vi "2015 Filepath Network Variable.vi"(5 "Network Var Set":u8, 7 "Washer In":T3={"Appliance Details"={"FileVersionInfo"={"FileVersion"="", "ProductName"="", "InternalName"="", "CompanyName"="", "LegalCopyright"="", "FileDescription"=""}, "Dishwasher Info"={"Open Cup Weight (gm):"=0.0, "Auto Cup Weight (gm):"=0.0, "Detergent-Dish:"="", "Inlet Temperature-Dish:"="", "Cycle Mode-Dish:"="", "Unit Control-Dish:"="", "Manufacturer-Dish:"=""}, "Washer Info"={"Hot Water Temperature (Fahrenheit):"="", "Cold Water Temperature (Fahrenheit):"="", "Capacity (cu.ft):"=0.0, "Initial Cloth Weight:"=0.0, "Cloth Lot:"=0, "Model Family:"="", "Program Name:"="", "Cycle Selection:"="", "Wash Temperature:"="", "Rinse Temperature:"="", "Load Size:"=""}, "File Name Output Array"=[], "Calibration Output Array"=[], "Appliance Common"={"Engineer:"="", "Model Number:"="", "Serial Number:"="", "Comments:"="", "Station ID:"="", "Technician:"="", "TR Number:"="", "Lab ID:"="", "Voltage:"="", "Water Pressure (PSI):"="", "Test Date:"="", "Computer Name:"="", "IP Address:"="", "Ambient RH:"="", "Frequency:"="", "Build:"="", "Filename:"="", "Test Type:"="", "Load Run #:"=0, "Ambient Temperature (F):"="", "File Path:"=path "", "Cycles Per Year"=60}, "Water Heater"={"Heating Mode:"=""}, "Dryer"={"Heat Setting:"="", "Washer Water Temperature (60 ± 5°F):"=60, "Water Hardness (PPM):"=17, "Dryness Setting:"="", "Dryer Type:"="", "Exhaust:"="", "Drying Cycle:"="", "Load Type:"="", "Nominal Load Weight"="", "Dryer Initial IMC Data"={"Measured IMC (lbs)"=7.0, "Actual Initial RMC (%)"=7.0, "RMC (Desired %)"=100.0, "Bone Dry Wt(lbs)"=7.0, "Tolerance(%)"=5.0, "Actual Final RMC (%)"=7.0, "CEF (lbf/kWh)"=0.0, "Minimum Weight (lbf)"=0.0, "Average Weight (lbf)"=0.0, "Maximum Weight (lbf)"=0.0, "Measured IMC In Range?"=FALSE, "Moisture Reduction Factor"=55.5, "Field Use Factor"=1.04, "Empty Dryer Cold Weigth"=0.0, "Energy Standard"=enum."D2-Automatic Dryer", "Weight Cloth (lbs)"=0.0, "Relative Moisture Content (%)"=0.0, "Relative Moisture Content - Avg (%)"=0.0}}}, "Display Data (RLT)"={"Status Color"=0, "Serial Number Display"="", "Cycle Count Display"=0, "Station Label Display"="", "Current Run Start Time Display"=0.0, "Board ID Display"="", "RPM Display"=0, "Current Display"=0.0, "Current Path Display"=path "", "Saving Display"=FALSE, "Unit Type Display"=enum."", "Total Time On Display"=0.0, "UI Button"=FALSE}} {"Display Data (RLT)"."Current Display" format="%.2f"; "Display Data (RLT)"."Cycle Count Display" format="%04d"; "Appliance Details"."Dryer"."Dryer Initial IMC Data"."Maximum Weight (lbf)" format="%03_6g"; "Appliance Details"."Dryer"."Dryer Initial IMC Data"."Average Weight (lbf)" format="%03_6g"; "Appliance Details"."Dryer"."Dryer Initial IMC Data"."Minimum Weight (lbf)" format="%03_6g"; "Appliance Details"."Dryer"."Dryer Initial IMC Data"."CEF (lbf/kWh)" format="%03_6g"; "Appliance Details"."Dryer"."Dryer Initial IMC Data"."Actual Final RMC (%)" format="%03_6g"; "Appliance Details"."Dryer"."Dryer Initial IMC Data"."Tolerance(%)" format="%0#_6g"; "Appliance Details"."Dryer"."Dryer Initial IMC Data"."Bone Dry Wt(lbs)" format="%03_6g"; "Appliance Details"."Dryer"."Dryer Initial IMC Data"."RMC (Desired %)" format="%0#_6g"; "Appliance Details"."Dryer"."Dryer Initial IMC Data"."Actual Initial RMC (%)" format="%03_6g"; "Appliance Details"."Dryer"."Dryer Initial IMC Data"."Measured IMC (lbs)" format="%0#_6g"}, 8 "error in (no error)":errorcluster, 10 "Network Variable Location":i32, 11 "File Locations In":T1={"General Setup Paths"={"Calibration File Path"=path "", "DOE Capacity Path"=path "", "Data Folder Path"=path "", "RLT Backup Data Path"=path "", "Tool Base Path"=path "", "General Startup Config Path"=path "", "File Save Previous Run Path"=path "", "File Save Configuration Data Path"=path "C:/Newfi Exe/Newfi Exe Locations.ini"}, "Data File Paths"={"Data File Path"=path "", "Debug File Path"=path "", "Bus Log Path"=path "", "Current"=path "", "Summary"=path ""}, "New Summary Created"=FALSE, "Check Location Interval (Second)"=2}) -> (0 "error out":errorcluster, 3 "File Locations Out":T1={"General Setup Paths"={"Calibration File Path"=path "", "DOE Capacity Path"=path "", "Data Folder Path"=path "", "RLT Backup Data Path"=path "", "Tool Base Path"=path "", "General Startup Config Path"=path "", "File Save Previous Run Path"=path "", "File Save Configuration Data Path"=path "C:/Newfi Exe/Newfi Exe Locations.ini"}, "Data File Paths"={"Data File Path"=path "", "Debug File Path"=path "", "Bus Log Path"=path "", "Current"=path "", "Summary"=path ""}, "New Summary Created"=FALSE, "Check Location Interval (Second)"=2})   [LabVIEW 2016]
uses:
  Utility/Save File/Public/Type Definitions/Save File Washer.ctl
  Utility/Save File/File Setup (Public)/Type Definition/Save File DISH Dishwasher Details.ctl
  <vilib>/Platform/fileVersionInfo.llb/FileVersionInformation.ctl
  Washer DOE/Type Definitions/DOE Appliance Common.ctl
  Utility/Custom Pallet Controls/Custom Pallet String.ctl
  Utility/Save File/File Setup (Public)/Type Definition/DPT IMC Data.ctl
  Washer DOE/Type Definitions/DOE Dryer Standard.ctl
  Utility/Save File/Public/Type Definitions/Save File Appliance Display.ctl
  Utility/Save File/Public/Type Definitions/Save File Unit Type.ctl
  Utility/Save File/File Setup (Public)/Type Definition/Save File DOE File Path Control.ctl
  Utility/Save File/File Setup (Public)/Type Definition/Save File DOE Data Save Filepaths.ctl
  Utility/Save File/Save File.lvlib
  Utility/Save File/File Setup.lvlib
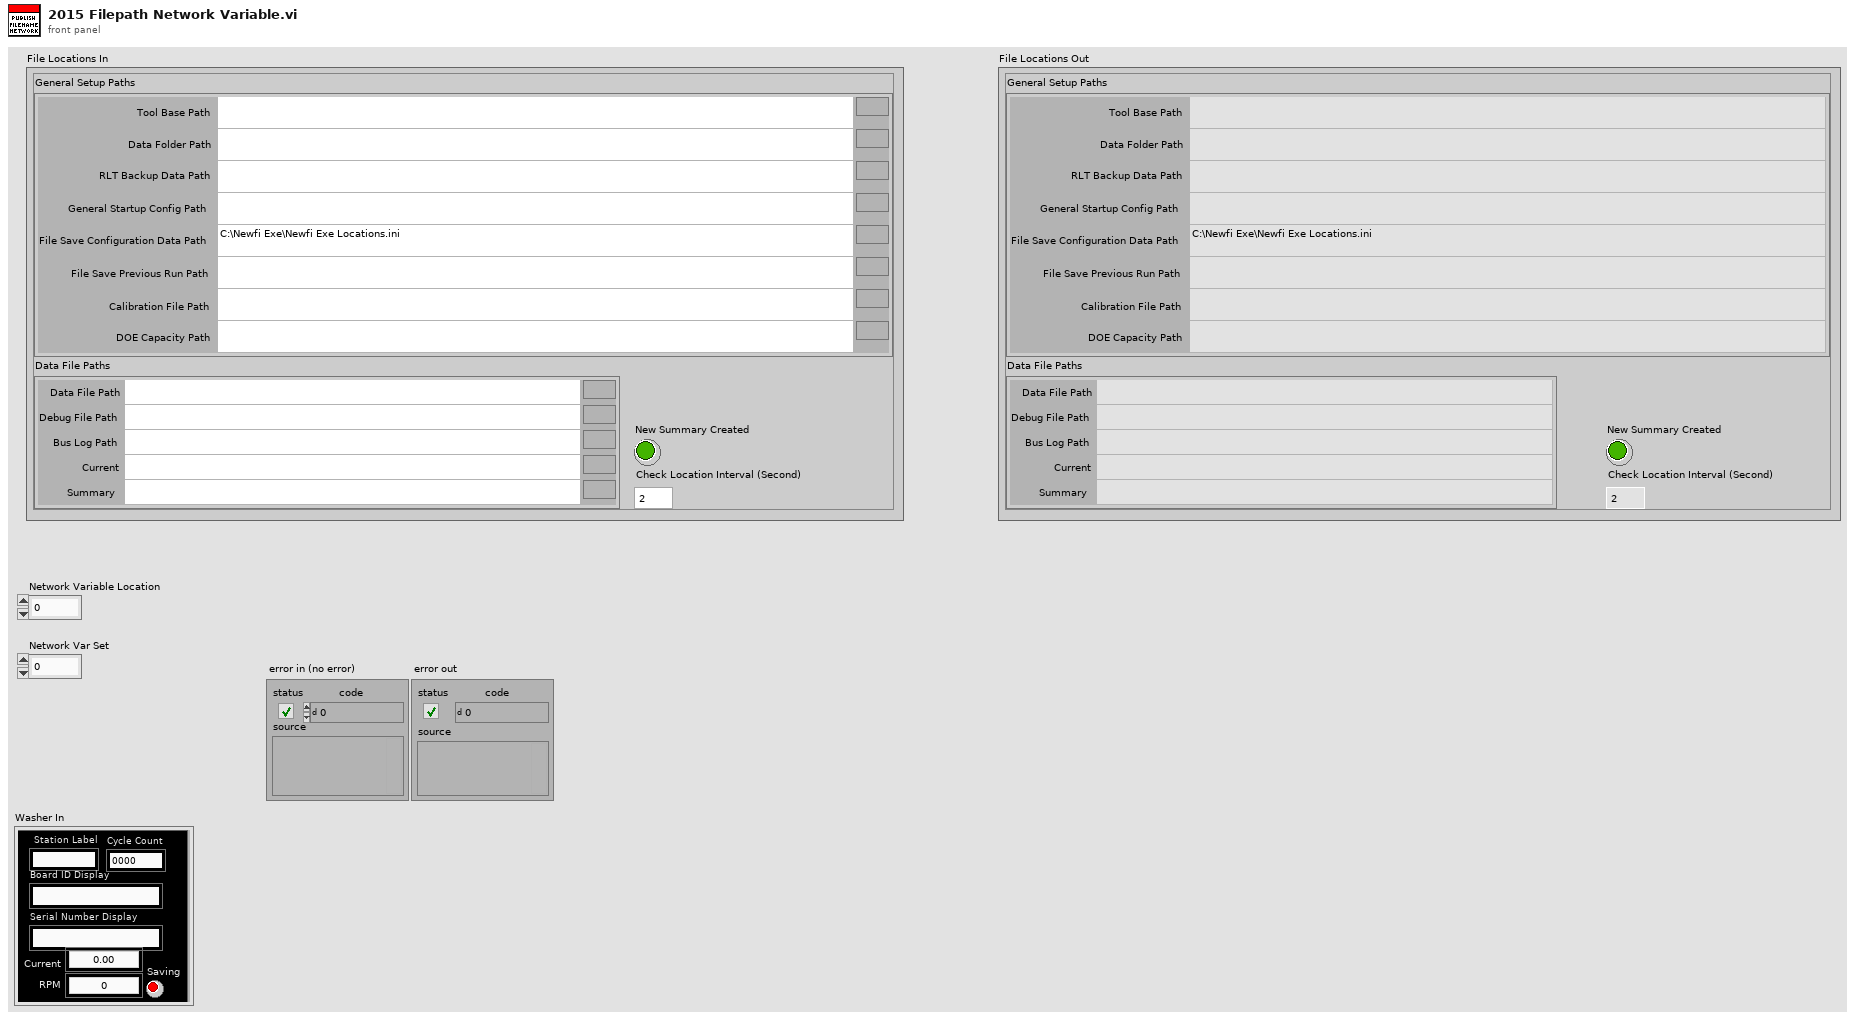
[diagram p1: front panel]
types:
  T1 = typedef "File Setup.lvlib/Save File DOE File Path Control.ctl" = cluster{"General Setup Paths":cluster{"Calibration File Path":path, "DOE Capacity Path":path, "Data Folder Path":path, "RLT Backup Data Path":path, "Tool Base Path":path, "General Startup Config Path":path, "File Save Previous Run Path":path, "File Save Configuration Data Path":path}, "Data File Paths":T2, "New Summary Created":bool, "Check Location Interval (Second)":i32}
  T2 = typedef "File Setup.lvlib/Save File DOE Data Save Filepaths.ctl" = cluster{"Data File Path":path, "Debug File Path":path, "Bus Log Path":path, "Current":path, "Summary":path}
  T3 = typedef "Save File.lvlib/Save File Washer.ctl" = cluster{"Appliance Details":T4, "Display Data (RLT)":T10}
  T4 = typedef "File Setup.lvlib/Save File DISH Dishwasher Details.ctl" = cluster{"FileVersionInfo":T5, "Dishwasher Info":cluster{"Open Cup Weight (gm):":dbl, "Auto Cup Weight (gm):":dbl, "Detergent-Dish:":string, "Inlet Temperature-Dish:":string, "Cycle Mode-Dish:":string, "Unit Control-Dish:":string, "Manufacturer-Dish:":string}, "Washer Info":cluster{"Hot Water Temperature (Fahrenheit):":string, "Cold Water Temperature (Fahrenheit):":string, "Capacity (cu.ft):":dbl, "Initial Cloth Weight:":dbl, "Cloth Lot:":i32, "Model Family:":string, "Program Name:":string, "Cycle Selection:":string, "Wash Temperature:":string, "Rinse Temperature:":string, "Load Size:":string}, "File Name Output Array":string[][], "Calibration Output Array":string[][], "Appliance Common":T6, "Water Heater":cluster{"Heating Mode:":string}, "Dryer":cluster{"Heat Setting:":T7, "Washer Water Temperature (60 ± 5°F):":u16, "Water Hardness (PPM):":u16, "Dryness Setting:":T7, "Dryer Type:":string, "Exhaust:":string, "Drying Cycle:":string, "Load Type:":string, "Nominal Load Weight":string, "Dryer Initial IMC Data":T8}}
  T5 = typedef "FileVersionInformation.ctl" = cluster{"FileVersion":string, "ProductName":string, "InternalName":string, "CompanyName":string, "LegalCopyright":string, "FileDescription":string}
  T6 = typedef "DOE Appliance Common.ctl" = cluster{"Engineer:":string, "Model Number:":string, "Serial Number:":string, "Comments:":string, "Station ID:":string, "Technician:":string, "TR Number:":string, "Lab ID:":string, "Voltage:":string, "Water Pressure (PSI):":string, "Test Date:":string, "Computer Name:":string, "IP Address:":string, "Ambient RH:":string, "Frequency:":string, "Build:":string, "Filename:":string, "Test Type:":string, "Load Run #:":i32, "Ambient Temperature (F):":string, "File Path:":path, "Cycles Per Year":u32}
  T7 = typedef "Custom Pallet String.ctl" = string
  T8 = typedef "DPT IMC Data.ctl" = cluster{"Measured IMC (lbs)":dbl, "Actual Initial RMC (%)":dbl, "RMC (Desired %)":dbl, "Bone Dry Wt(lbs)":dbl, "Tolerance(%)":dbl, "Actual Final RMC (%)":dbl, "CEF (lbf/kWh)":dbl, "Minimum Weight (lbf)":dbl, "Average Weight (lbf)":dbl, "Maximum Weight (lbf)":dbl, "Measured IMC In Range?":bool, "Moisture Reduction Factor":dbl, "Field Use Factor":dbl, "Empty Dryer Cold Weigth":dbl, "Energy Standard":T9, "Weight Cloth (lbs)":dbl, "Relative Moisture Content (%)":dbl, "Relative Moisture Content - Avg (%)":dbl}
  T9 = typedef "DOE Dryer Standard.ctl" = enum16{"D2-Automatic Dryer", "D2-Timer Dryer", "D1-Automatic Dryer", "D1-Timer Dryer", "Other"}
  T10 = typedef "Save File Appliance Display.ctl" = cluster{"Status Color":u32, "Serial Number Display":string, "Cycle Count Display":i32, "Station Label Display":string, "Current Run Start Time Display":dbl, "Board ID Display":string, "RPM Display":u32, "Current Display":dbl, "Current Path Display":path, "Saving Display":bool, "Unit Type Display":T11, "Total Time On Display":dbl, "UI Button":bool}
  T11 = typedef "Save File.lvlib/Save File Unit Type.ctl" = enum32{"", "Viper", "Hawk", "2015"}
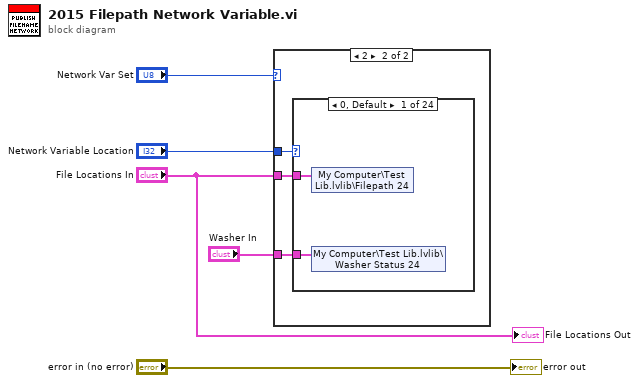
[diagram p0: block diagram]
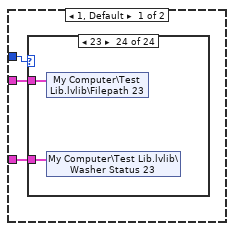
[diagram p2: hidden frame]
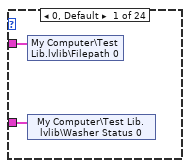
[diagram p3: hidden frame]
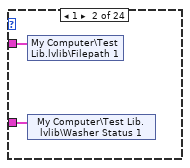
[diagram p4: hidden frame]
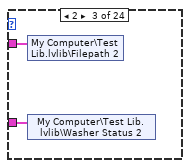
[diagram p5: hidden frame]
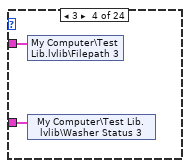
[diagram p6: hidden frame]
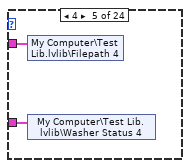
[diagram p7: hidden frame]
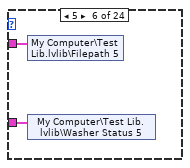
[diagram p8: hidden frame]
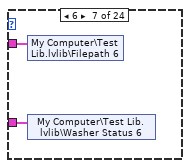
[diagram p9: hidden frame]
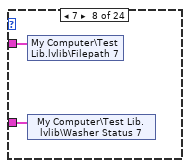
[diagram p10: hidden frame]
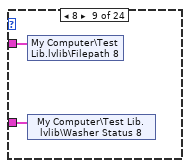
[diagram p11: hidden frame]
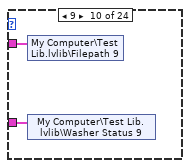
[diagram p12: hidden frame]
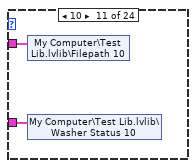
[diagram p13: hidden frame]
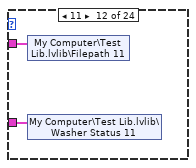
[diagram p14: hidden frame]
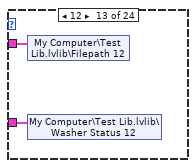
[diagram p15: hidden frame]
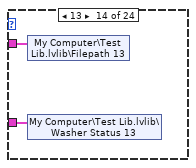
[diagram p16: hidden frame]
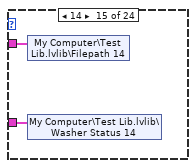
[diagram p17: hidden frame]
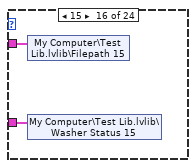
[diagram p18: hidden frame]
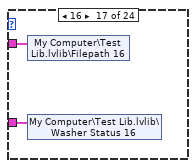
[diagram p19: hidden frame]
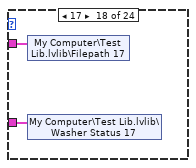
[diagram p20: hidden frame]
diagram:
  n1 = case shown="2" "Network Var Set" {
    tunnel: "File Locations In" -> [w8 w58]
    tunnel: "Network Variable Location" -> [w7 w57]
    tunnel: "Washer In" -> [w6 w59]
    frame 1, Default {
      n2 = case shown="23" w7 {
        tunnel: w8 -> [w10 w12 w14 w16 w18 w20 w22 w24 w26 w28 w30 w32 w34 w36 w38 w40 w42 w44 w46 w48 w50 w52 w54 w56]
        tunnel: w6 -> [w9 w11 w13 w15 w17 w19 w21 w23 w25 w27 w29 w31 w33 w35 w37 w39 w41 w43 w45 w47 w49 w51 w53 w55]
        frame 0, Default {
          n3 = shared-variable "My Computer\\Test Lib.lvlib\\Filepath 0"(w10) -> ()  [unwired: 1 in, 1 out]
          n4 = shared-variable "My Computer\\Test Lib.lvlib\\Washer Status 0"(w9) -> ()  [unwired: 1 in, 1 out]
        }
        frame 1 {
          n5 = shared-variable "My Computer\\Test Lib.lvlib\\Filepath 1"(w12) -> ()  [unwired: 1 in, 1 out]
          n6 = shared-variable "My Computer\\Test Lib.lvlib\\Washer Status 1"(w11) -> ()  [unwired: 1 in, 1 out]
        }
        frame 2 {
          n7 = shared-variable "My Computer\\Test Lib.lvlib\\Filepath 2"(w14) -> ()  [unwired: 1 in, 1 out]
          n8 = shared-variable "My Computer\\Test Lib.lvlib\\Washer Status 2"(w13) -> ()  [unwired: 1 in, 1 out]
        }
        frame 3 {
          n9 = shared-variable "My Computer\\Test Lib.lvlib\\Filepath 3"(w16) -> ()  [unwired: 1 in, 1 out]
          n10 = shared-variable "My Computer\\Test Lib.lvlib\\Washer Status 3"(w15) -> ()  [unwired: 1 in, 1 out]
        }
        frame 4 {
          n11 = shared-variable "My Computer\\Test Lib.lvlib\\Filepath 4"(w18) -> ()  [unwired: 1 in, 1 out]
          n12 = shared-variable "My Computer\\Test Lib.lvlib\\Washer Status 4"(w17) -> ()  [unwired: 1 in, 1 out]
        }
        frame 5 {
          n13 = shared-variable "My Computer\\Test Lib.lvlib\\Filepath 5"(w20) -> ()  [unwired: 1 in, 1 out]
          n14 = shared-variable "My Computer\\Test Lib.lvlib\\Washer Status 5"(w19) -> ()  [unwired: 1 in, 1 out]
        }
        frame 6 {
          n15 = shared-variable "My Computer\\Test Lib.lvlib\\Filepath 6"(w22) -> ()  [unwired: 1 in, 1 out]
          n16 = shared-variable "My Computer\\Test Lib.lvlib\\Washer Status 6"(w21) -> ()  [unwired: 1 in, 1 out]
        }
        frame 7 {
          n17 = shared-variable "My Computer\\Test Lib.lvlib\\Filepath 7"(w24) -> ()  [unwired: 1 in, 1 out]
          n18 = shared-variable "My Computer\\Test Lib.lvlib\\Washer Status 7"(w23) -> ()  [unwired: 1 in, 1 out]
        }
        frame 8 {
          n19 = shared-variable "My Computer\\Test Lib.lvlib\\Filepath 8"(w26) -> ()  [unwired: 1 in, 1 out]
          n20 = shared-variable "My Computer\\Test Lib.lvlib\\Washer Status 8"(w25) -> ()  [unwired: 1 in, 1 out]
        }
        frame 9 {
          n21 = shared-variable "My Computer\\Test Lib.lvlib\\Filepath 9"(w28) -> ()  [unwired: 1 in, 1 out]
          n22 = shared-variable "My Computer\\Test Lib.lvlib\\Washer Status 9"(w27) -> ()  [unwired: 1 in, 1 out]
        }
        frame 10 {
          n23 = shared-variable "My Computer\\Test Lib.lvlib\\Filepath 10"(w30) -> ()  [unwired: 1 in, 1 out]
          n24 = shared-variable "My Computer\\Test Lib.lvlib\\Washer Status 10"(w29) -> ()  [unwired: 1 in, 1 out]
        }
        frame 11 {
          n25 = shared-variable "My Computer\\Test Lib.lvlib\\Filepath 11"(w32) -> ()  [unwired: 1 in, 1 out]
          n26 = shared-variable "My Computer\\Test Lib.lvlib\\Washer Status 11"(w31) -> ()  [unwired: 1 in, 1 out]
        }
        frame 12 {
          n27 = shared-variable "My Computer\\Test Lib.lvlib\\Filepath 12"(w34) -> ()  [unwired: 1 in, 1 out]
          n28 = shared-variable "My Computer\\Test Lib.lvlib\\Washer Status 12"(w33) -> ()  [unwired: 1 in, 1 out]
        }
        frame 13 {
          n29 = shared-variable "My Computer\\Test Lib.lvlib\\Filepath 13"(w36) -> ()  [unwired: 1 in, 1 out]
          n30 = shared-variable "My Computer\\Test Lib.lvlib\\Washer Status 13"(w35) -> ()  [unwired: 1 in, 1 out]
        }
        frame 14 {
          n31 = shared-variable "My Computer\\Test Lib.lvlib\\Filepath 14"(w38) -> ()  [unwired: 1 in, 1 out]
          n32 = shared-variable "My Computer\\Test Lib.lvlib\\Washer Status 14"(w37) -> ()  [unwired: 1 in, 1 out]
        }
        frame 15 {
          n33 = shared-variable "My Computer\\Test Lib.lvlib\\Filepath 15"(w40) -> ()  [unwired: 1 in, 1 out]
          n34 = shared-variable "My Computer\\Test Lib.lvlib\\Washer Status 15"(w39) -> ()  [unwired: 1 in, 1 out]
        }
        frame 16 {
          n35 = shared-variable "My Computer\\Test Lib.lvlib\\Filepath 16"(w42) -> ()  [unwired: 1 in, 1 out]
          n36 = shared-variable "My Computer\\Test Lib.lvlib\\Washer Status 16"(w41) -> ()  [unwired: 1 in, 1 out]
        }
        frame 17 {
          n37 = shared-variable "My Computer\\Test Lib.lvlib\\Filepath 17"(w44) -> ()  [unwired: 1 in, 1 out]
          n38 = shared-variable "My Computer\\Test Lib.lvlib\\Washer Status 17"(w43) -> ()  [unwired: 1 in, 1 out]
        }
        frame 18 {
          n39 = shared-variable "My Computer\\Test Lib.lvlib\\Filepath 18"(w46) -> ()  [unwired: 1 in, 1 out]
          n40 = shared-variable "My Computer\\Test Lib.lvlib\\Washer Status 18"(w45) -> ()  [unwired: 1 in, 1 out]
        }
        frame 19 {
          n41 = shared-variable "My Computer\\Test Lib.lvlib\\Filepath 19"(w48) -> ()  [unwired: 1 in, 1 out]
          n42 = shared-variable "My Computer\\Test Lib.lvlib\\Washer Status 19"(w47) -> ()  [unwired: 1 in, 1 out]
        }
        frame 20 {
          n43 = shared-variable "My Computer\\Test Lib.lvlib\\Filepath 20"(w50) -> ()  [unwired: 1 in, 1 out]
          n44 = shared-variable "My Computer\\Test Lib.lvlib\\Washer Status 20"(w49) -> ()  [unwired: 1 in, 1 out]
        }
        frame 21 {
          n45 = shared-variable "My Computer\\Test Lib.lvlib\\Filepath 21"(w52) -> ()  [unwired: 1 in, 1 out]
          n46 = shared-variable "My Computer\\Test Lib.lvlib\\Washer Status 21"(w51) -> ()  [unwired: 1 in, 1 out]
        }
        frame 22 {
          n47 = shared-variable "My Computer\\Test Lib.lvlib\\Filepath 22"(w54) -> ()  [unwired: 1 in, 1 out]
          n48 = shared-variable "My Computer\\Test Lib.lvlib\\Washer Status 22"(w53) -> ()  [unwired: 1 in, 1 out]
        }
        frame 23 {
          n49 = shared-variable "My Computer\\Test Lib.lvlib\\Filepath 23"(w56) -> ()  [unwired: 1 in, 1 out]
          n50 = shared-variable "My Computer\\Test Lib.lvlib\\Washer Status 23"(w55) -> ()  [unwired: 1 in, 1 out]
        }
      }
    }
    frame 2 {
      n51 = case shown="0, Default" w57 {
        tunnel: w58 -> [w60 w63 w65 w67 w69 w70 w72 w75 w77 w79 w81 w83 w85 w86 w88 w91 w92 w95 w96 w98 w100 w103 w104 w106]
        tunnel: w59 -> [w61 w62 w64 w66 w68 w71 w73 w74 w76 w78 w80 w82 w84 w87 w89 w90 w93 w94 w97 w99 w101 w102 w105 w107]
        frame 0, Default {
          n52 = shared-variable "My Computer\\Test Lib.lvlib\\Filepath 24"(w60) -> ()  [unwired: 1 in, 1 out]
          n53 = shared-variable "My Computer\\Test Lib.lvlib\\Washer Status 24"(w61) -> ()  [unwired: 1 in, 1 out]
        }
        frame 1 {
          n54 = shared-variable "My Computer\\Test Lib.lvlib\\Filepath 25"(w63) -> ()  [unwired: 1 in, 1 out]
          n55 = shared-variable "My Computer\\Test Lib.lvlib\\Washer Status 25"(w62) -> ()  [unwired: 1 in, 1 out]
        }
        frame 2 {
          n56 = shared-variable "My Computer\\Test Lib.lvlib\\Filepath 26"(w65) -> ()  [unwired: 1 in, 1 out]
          n57 = shared-variable "My Computer\\Test Lib.lvlib\\Washer Status 26"(w64) -> ()  [unwired: 1 in, 1 out]
        }
        frame 3 {
          n58 = shared-variable "My Computer\\Test Lib.lvlib\\Filepath 27"(w67) -> ()  [unwired: 1 in, 1 out]
          n59 = shared-variable "My Computer\\Test Lib.lvlib\\Washer Status 27"(w66) -> ()  [unwired: 1 in, 1 out]
        }
        frame 4 {
          n60 = shared-variable "My Computer\\Test Lib.lvlib\\Filepath 28"(w69) -> ()  [unwired: 1 in, 1 out]
          n61 = shared-variable "My Computer\\Test Lib.lvlib\\Washer Status 28"(w68) -> ()  [unwired: 1 in, 1 out]
        }
        frame 5 {
          n62 = shared-variable "My Computer\\Test Lib.lvlib\\Filepath 29"(w70) -> ()  [unwired: 1 in, 1 out]
          n63 = shared-variable "My Computer\\Test Lib.lvlib\\Washer Status 29"(w71) -> ()  [unwired: 1 in, 1 out]
        }
        frame 6 {
          n64 = shared-variable "My Computer\\Test Lib.lvlib\\Filepath 30"(w72) -> ()  [unwired: 1 in, 1 out]
          n65 = shared-variable "My Computer\\Test Lib.lvlib\\Washer Status 30"(w73) -> ()  [unwired: 1 in, 1 out]
        }
        frame 7 {
          n66 = shared-variable "My Computer\\Test Lib.lvlib\\Filepath 31"(w75) -> ()  [unwired: 1 in, 1 out]
          n67 = shared-variable "My Computer\\Test Lib.lvlib\\Washer Status 31"(w74) -> ()  [unwired: 1 in, 1 out]
        }
        frame 8 {
          n68 = shared-variable "My Computer\\Test Lib.lvlib\\Filepath 32"(w77) -> ()  [unwired: 1 in, 1 out]
          n69 = shared-variable "My Computer\\Test Lib.lvlib\\Washer Status 32"(w76) -> ()  [unwired: 1 in, 1 out]
        }
        frame 9 {
          n70 = shared-variable "My Computer\\Test Lib.lvlib\\Filepath 33"(w79) -> ()  [unwired: 1 in, 1 out]
          n71 = shared-variable "My Computer\\Test Lib.lvlib\\Washer Status 33"(w78) -> ()  [unwired: 1 in, 1 out]
        }
        frame 10 {
          n72 = shared-variable "My Computer\\Test Lib.lvlib\\Filepath 34"(w81) -> ()  [unwired: 1 in, 1 out]
          n73 = shared-variable "My Computer\\Test Lib.lvlib\\Washer Status 34"(w80) -> ()  [unwired: 1 in, 1 out]
        }
        frame 11 {
          n74 = shared-variable "My Computer\\Test Lib.lvlib\\Filepath 35"(w83) -> ()  [unwired: 1 in, 1 out]
          n75 = shared-variable "My Computer\\Test Lib.lvlib\\Washer Status 35"(w82) -> ()  [unwired: 1 in, 1 out]
        }
        frame 12 {
          n76 = shared-variable "My Computer\\Test Lib.lvlib\\Filepath 36"(w85) -> ()  [unwired: 1 in, 1 out]
          n77 = shared-variable "My Computer\\Test Lib.lvlib\\Washer Status 36"(w84) -> ()  [unwired: 1 in, 1 out]
        }
        frame 13 {
          n78 = shared-variable "My Computer\\Test Lib.lvlib\\Filepath 37"(w86) -> ()  [unwired: 1 in, 1 out]
          n79 = shared-variable "My Computer\\Test Lib.lvlib\\Washer Status 37"(w87) -> ()  [unwired: 1 in, 1 out]
        }
        frame 14 {
          n80 = shared-variable "My Computer\\Test Lib.lvlib\\Filepath 38"(w88) -> ()  [unwired: 1 in, 1 out]
          n81 = shared-variable "My Computer\\Test Lib.lvlib\\Washer Status 38"(w89) -> ()  [unwired: 1 in, 1 out]
        }
        frame 15 {
          n82 = shared-variable "My Computer\\Test Lib.lvlib\\Filepath 39"(w91) -> ()  [unwired: 1 in, 1 out]
          n83 = shared-variable "My Computer\\Test Lib.lvlib\\Washer Status 39"(w90) -> ()  [unwired: 1 in, 1 out]
        }
        frame 16 {
          n84 = shared-variable "My Computer\\Test Lib.lvlib\\Filepath 40"(w92) -> ()  [unwired: 1 in, 1 out]
          n85 = shared-variable "My Computer\\Test Lib.lvlib\\Washer Status 40"(w93) -> ()  [unwired: 1 in, 1 out]
        }
        frame 17 {
          n86 = shared-variable "My Computer\\Test Lib.lvlib\\Filepath 41"(w95) -> ()  [unwired: 1 in, 1 out]
          n87 = shared-variable "My Computer\\Test Lib.lvlib\\Washer Status 41"(w94) -> ()  [unwired: 1 in, 1 out]
        }
        frame 18 {
          n88 = shared-variable "My Computer\\Test Lib.lvlib\\Filepath 42"(w96) -> ()  [unwired: 1 in, 1 out]
          n89 = shared-variable "My Computer\\Test Lib.lvlib\\Washer Status 42"(w97) -> ()  [unwired: 1 in, 1 out]
        }
        frame 19 {
          n90 = shared-variable "My Computer\\Test Lib.lvlib\\Filepath 43"(w98) -> ()  [unwired: 1 in, 1 out]
          n91 = shared-variable "My Computer\\Test Lib.lvlib\\Washer Status 43"(w99) -> ()  [unwired: 1 in, 1 out]
        }
        frame 20 {
          n92 = shared-variable "My Computer\\Test Lib.lvlib\\Filepath 44"(w100) -> ()  [unwired: 1 in, 1 out]
          n93 = shared-variable "My Computer\\Test Lib.lvlib\\Washer Status 44"(w101) -> ()  [unwired: 1 in, 1 out]
        }
        frame 21 {
          n94 = shared-variable "My Computer\\Test Lib.lvlib\\Filepath 45"(w103) -> ()  [unwired: 1 in, 1 out]
          n95 = shared-variable "My Computer\\Test Lib.lvlib\\Washer Status 45"(w102) -> ()  [unwired: 1 in, 1 out]
        }
        frame 22 {
          n96 = shared-variable "My Computer\\Test Lib.lvlib\\Filepath 46"(w104) -> ()  [unwired: 1 in, 1 out]
          n97 = shared-variable "My Computer\\Test Lib.lvlib\\Washer Status 46"(w105) -> ()  [unwired: 1 in, 1 out]
        }
        frame 23 {
          n98 = shared-variable "My Computer\\Test Lib.lvlib\\Filepath 47"(w106) -> ()  [unwired: 1 in, 1 out]
          n99 = shared-variable "My Computer\\Test Lib.lvlib\\Washer Status 47"(w107) -> ()  [unwired: 1 in, 1 out]
        }
      }
    }
  }
  "error out" <- "error in (no error)"
  "File Locations Out" <- "File Locations In"
